vi "programa 3 adicion de datos a un archivo de texto.vi"() -> ()   [LabVIEW 2011]
panel:
  out "Array":dbl[](array[numeric])
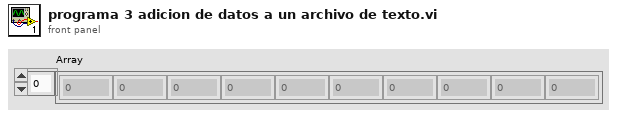
[diagram p1: front panel]
types:
  T1 = enum16{"open", "replace", "create", "open or create", "replace or create", "replace or create with confirmation"}
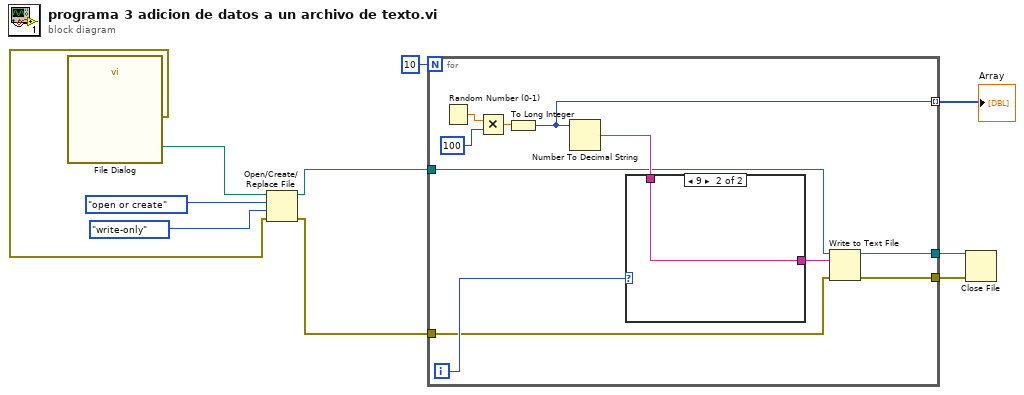
[diagram p0: block diagram]
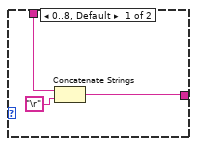
[diagram p2: hidden frame]
diagram:
  n1 = call "File Dialog"() -> ("selected path"=w10:path, "error out"=w9:errorcluster)  [unwired: 12 in, 2 out]
  n2 = Open/Create/Replace File(file path (use dialog)=w10, error in=w9, operation (0:open)=T1."open or create", access (0:read/write)=enum16{"read/write", "read-only", "write-only"}."write-only") -> (refnum out=w5:refnum<file>, error out=w4:errorcluster)  [unwired: 2 in, 1 out]
  n3 = for {
    N: 10 -> [_]
    tunnel: w5 -> [w15]
    tunnel: w4 -> [w14]
    tunnel: [w13] -> w3 mode=indexing
    tunnel: [w12] -> w2
    tunnel: [w11] -> w1
    i -> [w16]
    n4 = Random Number (0-1)() -> (number: 0 to 1=w21:dbl)
    n5 = Multiply(x=w21, y=100) -> (x*y=w19:dbl)
    n6 = To Long Integer(number=w19) -> (32bit integer=w13:i32)
    n7 = Number To Decimal String(number=w13) -> (decimal integer string=w18:string)  [unwired: 1 in]
    n8 = case shown="9" w16 {
      tunnel: w18 -> [w23 w25]
      tunnel: [w22 w25] -> w17
      frame 0..8, Default {
        n9 = Concatenate Strings "Concatenate Strings"(w23, "\r") -> (w22:string)
      }
      frame 9 {
      }
    }
    n10 = Write to Text File(file (use dialog)=w15, text=w17, error in=w14) -> (refnum out=w12:refnum<file>, error out=w11:errorcluster)  [unwired: 1 in, 1 out]
  }
  "Array" <- w3
  n11 = Close File(refnum=w2, error in=w1) -> ()  [unwired: 2 out]
